vi "Element Type.vi"(11 "HtmlButtonControl in":refnum<class "HttpButtonControl.lvclass">) -> (2 "Element Type":string)   [LabVIEW 2020, in "VolatusGUIElements.lvlib" / "HttpButtonControl.lvclass"]
uses:
  HttpButtonControl.lvclass
  HttpButtonControl.lvclass/HttpButtonControl.ctl
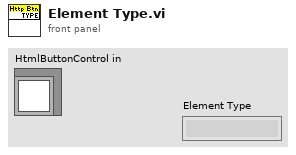
[diagram p1: front panel]
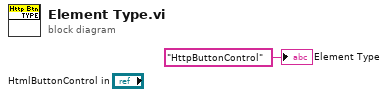
[diagram p0: block diagram]
diagram:
  "Element Type" <- "HttpButtonControl" ("Element Type")
